vi "Deadband Simulator.vi"(1 "死区(%)":dbl=1.0 format="%.2f", 3 "请求位置(%)":dbl format="%.2f") -> (0 "实际位置(%)":dbl format="%.2f")   [LabVIEW 2016]
doc: "仿真死区发生器。输出不变，直到输入至少大于或小于死区（单位百分比）。"
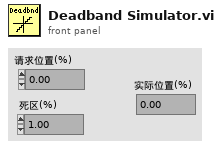
[diagram p1: front panel]
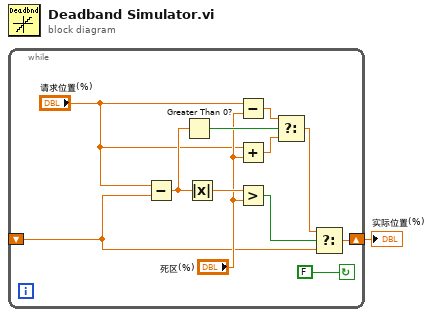
[diagram p0: block diagram]
diagram:
  n1 = while {
    shift-left: _ -> [w4]
    shift-right: [w11] -> w1
    stop <- FALSE continue-if-true
    n2 = Subtract(x="请求位置(%)", y=w4) -> (x-y=w10:dbl)
    n3 = Greater Than 0?(x=w10) -> (x > 0?=w9:bool)
    n4 = Absolute Value(x=w10) -> (abs(x)=w13:dbl)
    n5 = Subtract(x="请求位置(%)", y="死区(%)") -> (x-y=w5:dbl)
    n6 = Add(x="请求位置(%)", y="死区(%)") -> (x+y=w6:dbl)
    n7 = Greater?(x=w13, y="死区(%)") -> (0:w12:bool)
    n8 = Select(t=w5, s=w9, f=w6) -> (s? t:f=w3:dbl)
    n9 = Select(t=w3, s=w12, f=w4) -> (s? t:f=w11:dbl)
  }
  "实际位置(%)" <- w1
